vi "Write dev in px.vi"(8 "error in (no error)":errorcluster, 10 "dev in px":bool, 11 "Analyze BeamDeviation in":refnum<class "Analyze BeamDeviation.lvclass">) -> (0 "error out":errorcluster, 3 "Analyze BeamDeviation out":refnum<class "Analyze BeamDeviation.lvclass">)   [LabVIEW 2020, in "Analyze.lvlib" / "Analyze BeamDeviation.lvclass"]
uses:
  Analyze BeamDeviation.lvclass
  Analyze BeamDeviation.lvclass/Analyze BeamDeviation.ctl
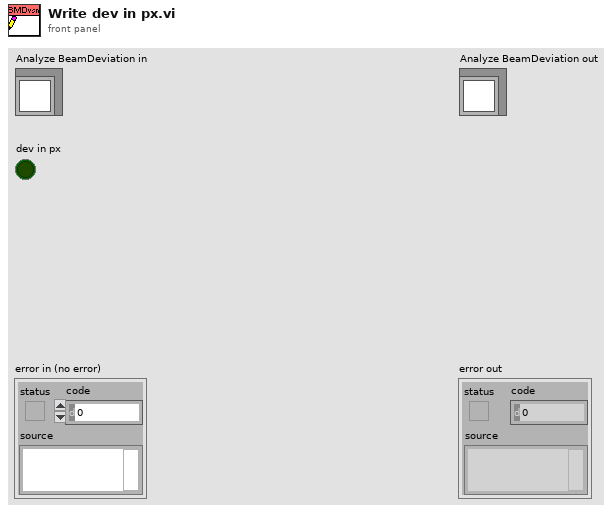
[diagram p1: front panel]
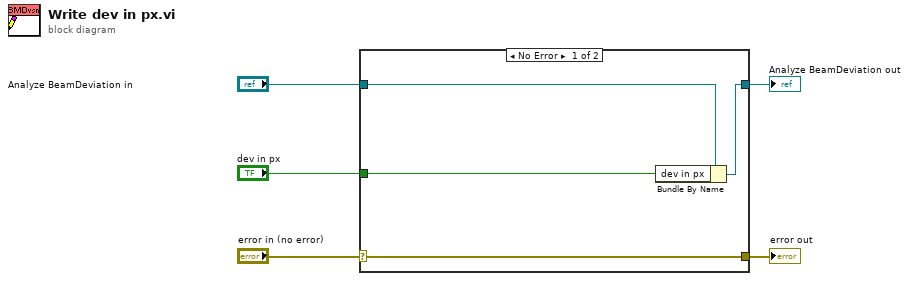
[diagram p0: block diagram]
diagram:
  n1 = case shown="No Error" "error in (no error)" {
    selector: "error in (no error)" -> [w9 w10]
    tunnel: [w9 w10] -> w4
    tunnel: [w7 w11] -> w2
    tunnel: "Analyze BeamDeviation in" -> [w8 w11]
    tunnel: "dev in px" -> [w6 _]
    frame No Error {
      n2 = Bundle By Name(cluster=w8, "dev in px"=w6) -> (w7:refnum<class "Analyze BeamDeviation.lvclass">)
    }
    frame Error {
    }
  }
  "error out" <- w4
  "Analyze BeamDeviation out" <- w2
